vi "REC_OptionalParameter.vi"(11 "Number":i32) -> (3 "String":string)   [LabVIEW 2020]
doc: "Transform number to string when larger then zero or return empty string otherwise."
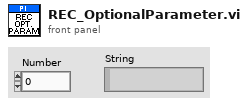
[diagram p1: front panel]
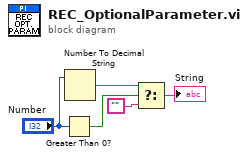
[diagram p0: block diagram]
diagram:
  n1 = Greater Than 0?(x="Number") -> (x > 0?=w3:bool)
  n2 = Number To Decimal String(number="Number") -> (decimal integer string=w1:string)  [unwired: 1 in]
  n3 = Select(t=w1, s=w3, f="") -> (s? t:f=→"String":string)
